vi "init_NI.vi"(6 "frame#":dbl, 7 "Piezol Signal":i32[](array[numeric]), 8 "flyback step#":dbl, 9 "one frame#":dbl, 11 "Galvo Signal":i32[](array[numeric])) -> (3 "output cluster":T1, 5 "actual number of samples written per channel":u32)   [LabVIEW 2015]
uses:
  <vilib>/DAQmx/write.llb/DAQmx Write (Analog 1D DBL 1Chan NSamp).vi
  <vilib>/DAQmx/write.llb/DAQmx Write (Digital 1D U32 1Chan NSamp).vi
  <vilib>/DAQmx/create/channels.llb/DAQmx Create Channel (DO-Digital Output).vi
  <vilib>/DAQmx/create/channels.llb/DAQmx Create Channel (AO-Voltage-Basic).vi
  <vilib>/DAQmx/configure/timing.llb/DAQmx Timing (Sample Clock).vi
  <vilib>/DAQmx/configure/trigger.llb/DAQmx Start Trigger (Digital Edge).vi
  <vilib>/DAQmx/miscellaneous.llb/DAQmx Fill In Error Info.vi
  <vilib>/DAQmx/create/channels.llb/DAQmx Create Channel (CO-Pulse Generation-Frequency).vi
  <vilib>/DAQmx/configure/timing.llb/DAQmx Timing (Implicit).vi
  <vilib>/DAQmx/create/channels.llb/DAQmx Create Channel (CO-Pulse Generation-Ticks).vi
  <resource>/objmgr/daqmx.rc
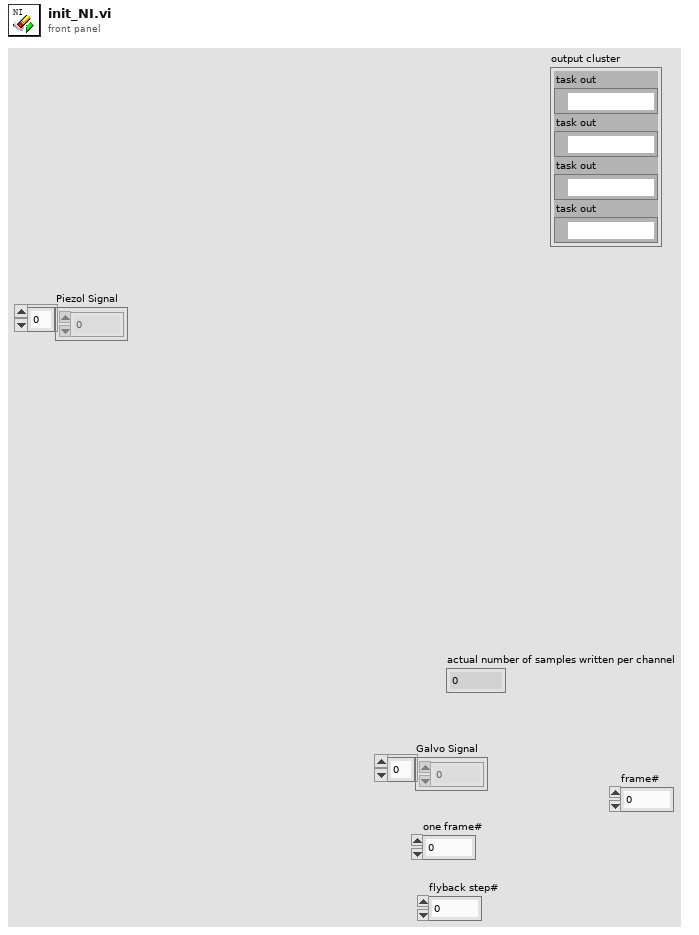
[diagram p1: front panel]
types:
  T1 = cluster{"task out":refnum<k21>, "task out":refnum<k21>, "task out":refnum<k21>, "task out":refnum<k21>}
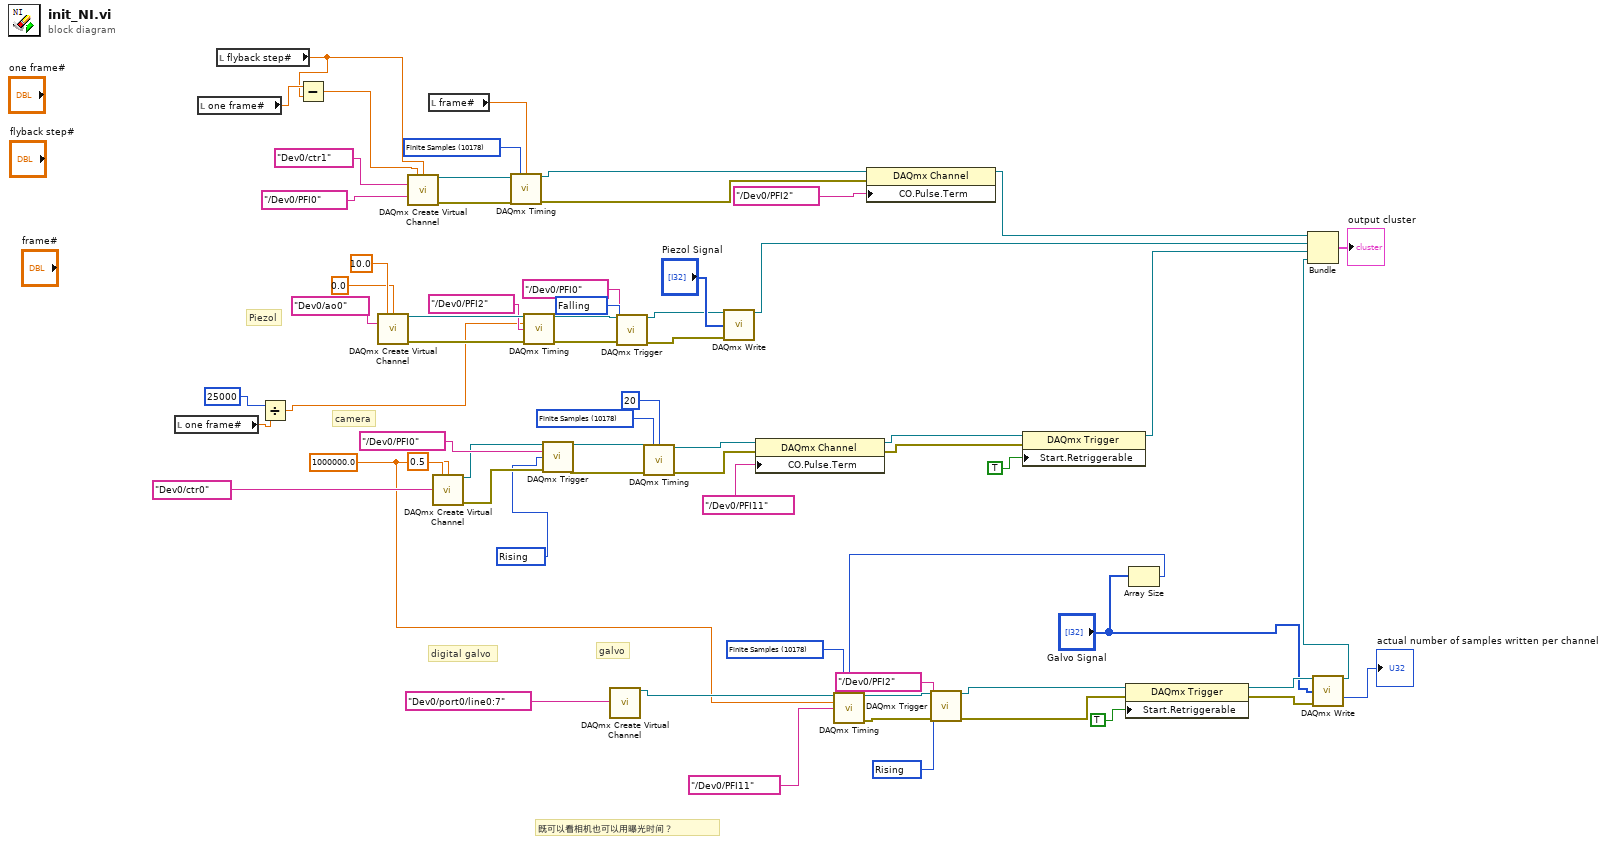
[diagram p0: block diagram]
diagram:
  w12 = 10171 items=["Rising"=10280, "Falling"=10171] ("edge")
  w23 = 1000000.0 ("frequency")
  w26 = 10178 items=["Finite Samples"=10178, "Continuous Samples"=10123, "Hardware Timed Single Point"=12522] ("sample mode")
  w44 = 10178 items=["Finite Samples"=10178, "Continuous Samples"=10123, "Hardware Timed Single Point"=12522] ("sample mode")
  w48 = 10280 items=["Rising"=10280, "Falling"=10171] ("edge")
  w61 = 10280 items=["Rising"=10280, "Falling"=10171] ("edge")
  w64 = 10178 items=["Finite Samples"=10178, "Continuous Samples"=10123, "Hardware Timed Single Point"=12522] ("sample mode")
  # "Piezol"
  # "camera"
  # "digital galvo"
  # "既可以看相机也可以用曝光时间？"
  # "galvo"
  n1 = local read "one frame#"() -> (w1:dbl)
  n2 = local read "one frame#"() -> (w4:dbl)
  n3 = local read "flyback step#"() -> (w3:dbl)
  n4 = Divide(x=25000, y=w1) -> (x/y=w10:dbl)
  n5 = Subtract(x=w4, y=w3) -> (x-y=w5:dbl)
  n6 = call-poly <vilib>:"DAQmx Create Virtual Channel.vi"("maximum value"=10.0, "minimum value"=0.0, "physical channels"=tag "Dev0/ao0") -> ("task out"=w29:refnum<k21>, "error out"=w28:errorcluster)  [unwired: 11 in]
  n7 = call-poly <vilib>:"DAQmx Create Virtual Channel.vi"("high ticks"=w5, "low ticks"=w3, "counter"=tag "Dev0/ctr1", "source of ticks"=tag "/Dev0/PFI0") -> ("task out"=w38:refnum<k21>, "error out"=w37:errorcluster)  [unwired: 10 in]
  n8 = local read "frame#"() -> (w25:dbl)
  n9 = call-poly <vilib>:"DAQmx Create Virtual Channel.vi"("frequency"=w23, "duty cycle"=0.5, "counter"=tag "Dev0/ctr0") -> ("task out"=w52:refnum<k21>, "error out"=w49:errorcluster)  [unwired: 11 in]
  n10 = call-poly <vilib>:"DAQmx Timing.vi"("task/channels in"=w38, "sample mode"=w26, "samples per channel"=w25, "error in"=w37) -> ("task out"=w35:refnum<k21>, "error out"=w34:errorcluster)  [unwired: 10 in]
  n11 = call-poly <vilib>:"DAQmx Timing.vi"("task/channels in"=w29, "rate"=w10, "source"=tag "/Dev0/PFI2", "error in"=w28) -> ("task out"=w16:refnum<k21>, "error out"=w15:errorcluster)  [unwired: 10 in]
  n12 = call-poly <vilib>:"DAQmx Trigger.vi"("task/channels in"=w52, "source"=tag "/Dev0/PFI0", "edge"=w48, "error in"=w49) -> ("task out"=w51:refnum<k21>, "error out"=w50:errorcluster)  [unwired: 10 in]
  n13 = call-poly <vilib>:"DAQmx Create Virtual Channel.vi"("lines"=tag "Dev0/port0/line0:7") -> ("task out"=w65:refnum<k21>)  [unwired: 13 in, 1 out]
  n14 = call-poly <vilib>:"DAQmx Trigger.vi"("task/channels in"=w16, "source"=tag "/Dev0/PFI0", "edge"=w12, "error in"=w15) -> ("task out"=w14:refnum<k21>, "error out"=w13:errorcluster)  [unwired: 10 in]
  n15 = call-poly <vilib>:"DAQmx Timing.vi"("task/channels in"=w51, "sample mode"=w44, "samples per channel"=20, "error in"=w50) -> ("task out"=w47:refnum<k21>, "error out"=w45:errorcluster)  [unwired: 10 in]
  n16 = call-poly <vilib>:"DAQmx Write.vi"("task/channels in"=w14, "data"="Piezol Signal", "error in"=w13) -> ("task out"=w20:refnum<k21>)  [unwired: 10 in, 2 out]
  n17 = property class="DAQmx Channel"(reference=w47, error in=w45, "CO.Pulse.Term"=tag "/Dev0/PFI11" ("source")) -> (reference out=w8:refnum<k21>, error out=w7:errorcluster)
  n18 = property class="DAQmx Channel"(reference=w35, error in=w34, "CO.Pulse.Term"=tag "/Dev0/PFI2") -> (reference out=w21:refnum<k21>)  [unwired: 1 out]
  n19 = property class="DAQmx Trigger"(reference=w8, error in=w7, "Start.Retriggerable"=TRUE) -> (reference out=w6:refnum<k21>)  [unwired: 1 out]
  n20 = Array Size(array="Galvo Signal") -> (size(s)=w41:i32)
  n21 = call-poly <vilib>:"DAQmx Timing.vi"("task/channels in"=w65, "sample mode"=w64, "samples per channel"=w41, "rate"=w23, "source"=tag "/Dev0/PFI11") -> ("task out"=w63:refnum<k21>, "error out"=w62:errorcluster)  [unwired: 9 in]
  n22 = call-poly <vilib>:"DAQmx Trigger.vi"("task/channels in"=w63, "source"=tag "/Dev0/PFI2", "edge"=w61, "error in"=w62) -> ("task out"=w57:refnum<k21>, "error out"=w56:errorcluster)  [unwired: 10 in]
  n23 = property class="DAQmx Trigger"(reference=w57, error in=w56, "Start.Retriggerable"=TRUE) -> (reference out=w58:refnum<k21>, error out=w59:errorcluster)
  n24 = call-poly <vilib>:"DAQmx Write.vi"("task/channels in"=w58, "data"="Galvo Signal", "error in"=w59) -> ("task out"=w19:refnum<k21>, "number of samples written per channel"=→"actual number of samples written per channel":u32)  [unwired: 10 in, 1 out]
  n25 = Bundle("task out"=w21, "task out"=w20, "task out"=w6, "task out"=w19) -> (→"output cluster":T1)  [unwired: 1 in]
